vi "Functions Scan.vi"(8 "error in (no error)":errorcluster, 11 "Controller in":refnum<class "Controller.lvclass">) -> (0 "error out":errorcluster, 3 "Controller out":refnum<class "Controller.lvclass">)   [LabVIEW 2016, in "Controller Actor.lvlib" / "Controller.lvclass"]
uses:
  <userlib>/Common Components/Controller/Controller.lvclass
  C:/Program Files (x86)/National Instruments/LabVIEW 2016/vi.lib/ActorFramework/Actor/Actor.lvclass
  <userlib>/Common Components/Controller/Controller.lvclass/Controller.ctl
  <vilib>/ActorFramework/Actor/Actor.lvclass/Actor.ctl
  <vilib>/ActorFramework/Message Enqueuer/Message Enqueuer.lvclass/Message Enqueuer.ctl
  <userlib>/Common Components/Controller/Accessors/Read Root Path.vi
  <vilib>/ActorFramework/Message Enqueuer/Init from Existing Queue.vi
  <vilib>/ActorFramework/Message Enqueuer/Message Enqueuer.lvclass
  <vilib>/ActorFramework/Actor/Actor.lvclass
  <userlib>/Common Components/Controller/Messages/Log Status/Log Status.lvclass
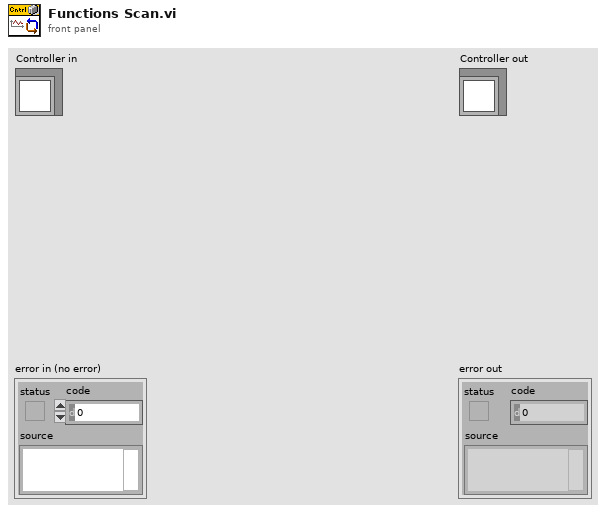
[diagram p1: front panel]
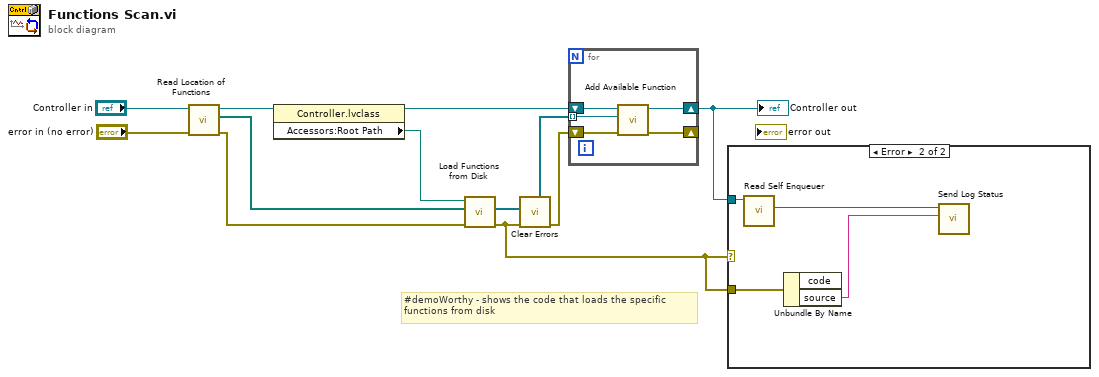
[diagram p0: block diagram]
diagram:
  # "#demoWorthy - shows the code that loads the specific\nfunctions from disk"
  n1 = call <userlib>:"Read Location of Functions.vi"("error in (no error)"="error in (no error)", "Controller in"="Controller in") -> ("error out"=w9:errorcluster, "Array of Function Location"=w8:path[], "Controller out"=w6:refnum<class "Controller.lvclass">)  [unwired: 7 in]
  n2 = property class="Controller.lvclass"(reference=w6) -> (reference out=w4:refnum<class "Controller.lvclass">, "Accessors:Root Path"=w5:path)  [unwired: 1 in, 1 out]
  n3 = call <userlib>:"Load Functions from Disk.vi"("error in (no error)"=w9, "Array of paths (folders to scan or explicit files)"=w8, "base path"=w5) -> ("error out"=w1:errorcluster, "Available Functions"=w7:refnum<class "Function.lvclass">[])  [unwired: 7 in]
  n4 = call <vilib>:"Clear Errors.vi"("error in (no error)"=w1) -> ("error out"=w2:errorcluster)  [unwired: 5 in, 1 out]
  n5 = for {
    tunnel: w7 -> [w14] mode=indexing
    shift-right: [w15] -> w3
    shift-left: w4 -> [w16]
    shift-right: [w12] -> _
    shift-left: w2 -> [w13]
    n6 = call <userlib>:"Add Available Function.vi"("error in (no error)"=w13, "Function.lvclass"=w14, "Controller in"=w16) -> ("error out"=w12:errorcluster, "Controller out"=w15:refnum<class "Controller.lvclass">)  [unwired: 7 in]
  }
  "Controller out" <- w3
  n7 = case shown="Error" w1 {
    tunnel: w3 -> [_ w20]
    tunnel: w1 -> [_ w18]
    frame No Error {
    }
    frame Error {
      n8 = call <vilib>:"Read Self Enqueuer.vi"("Actor"=w20) -> ("Self Enqueuer"=w19:refnum<class "Message Enqueuer.lvclass">)  [unwired: 10 in]
      n9 = Unbundle By Name(w18) -> ("source"=w17:string)  [unwired: 1 out]
      n10 = call <userlib>:"Send Log Status.vi"("String"=w17, "Message Enqueuer in"=w19) -> ()  [unwired: 8 in, 2 out]
    }
  }
